vi "Stop Core.vi"(10 "final error code":i32, 11 "Photometrics Camera in":refnum<class "Photometrics Camera.lvclass">) -> (3 "Photometrics Camera out":refnum<class "Photometrics Camera.lvclass">)   [LabVIEW 2018, in "Photometrics Camera.lvlib" / "Photometrics Camera.lvclass"]
doc: "(<B>Filename</B>: Actor Framework.lvlib:Actor.lvclass:Stop Core.vi)\n\nDefines what the actor does before it stops. Use the <B>final error code</B> input to determine whether the actor shut down in response to an error.\n\nBy default, this method does nothing. A descendant class may override it to define behavior, such as shutting down any processes the actor initiated in its override of the Actor Core method."
uses:
  Photometrics Camera.lvclass
  C:/FlashGordon/Development/dll/PVCamNET.dll
  Development/dll/PVCamNET.dll
  Camera/Camera.lvclass
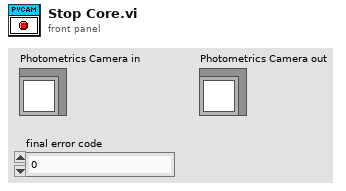
[diagram p1: front panel]
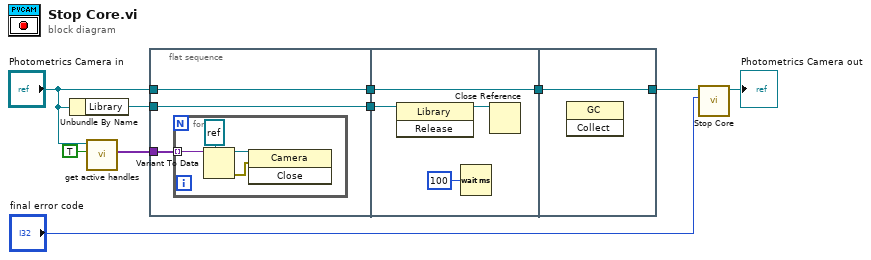
[diagram p0: block diagram]
diagram:
  n1 = Unbundle By Name("Photometrics Camera in") -> ("Library"=w7:refnum<k24>)
  n2 = call-dynamic "get active handles.vi"("Return All?"=TRUE, "Camera in"="Photometrics Camera in") -> ("Handles"=w1:variant[])  [unwired: 5 in, 4 out]
  n3 = flat-sequence {
    tunnel: w7 -> [w12]
    tunnel: "Photometrics Camera in" -> [w13]
    tunnel: [w13] -> w6
    tunnel: [w12] -> w5
    tunnel: w1 -> [w11]
    tunnel: [w19] -> w8
    tunnel: w6 -> [w19]
    tunnel: w5 -> [w18]
    tunnel: [w22] -> w4
    tunnel: w8 -> [w22]
    frame #0 {
      n4 = for {
        tunnel: w11 -> [w17] mode=indexing
        n5 = Variant To Data(type=refnum<k24> refnum ("reference out"), Variant=w17) -> (data=w16:refnum<k24>, error out=w15:errorcluster)  [unwired: 1 in]
        n6 = invoke class="Camera" method="Close"(reference=w16, error in=w15) -> ()  [unwired: 1 in, 3 out]
      }
    }
    frame #1 {
      n7 = invoke class="Library" method="Release"(reference=w18) -> (reference out=w21:refnum<k24>)  [unwired: 2 in, 2 out]
      n8 = Wait (ms)(milliseconds to wait=u32 100) -> ()  [unwired: 1 out]
      n9 = Close Reference(reference=w21) -> ()  [unwired: 1 in, 1 out]
    }
    frame #2 {
      n10 = invoke class="GC" method="Collect"() -> ()  [unwired: 3 in, 3 out]
    }
  }
  n11 = call-parent "Stop Core.vi"("final error code"="final error code", "Device in"=w4) -> ("Device out"=→"Photometrics Camera out":refnum<class "Photometrics Camera.lvclass">)  [unwired: 9 in]
